vi "FT10_Fornax Power Down.vi"(10 "Auto Set Power Cluster in":T1, 11 "Message Handling Cluster in":T5={"Fornax Connected?"=refnum, "Unitherm Connected?"=refnum, "M4X Connected?"=refnum, "Unitherm Connect/Disconnect"=refnum, "Fornax Connection"=refnum, "UNITHERM Connection"="", "M4X Connection"=0, "FPGA VI Reference Out"=refnum, "PXI-7854R Connected?"=refnum, "Fornax Connect/Disconnect"=refnum, "7854 Connect/Disconnect"=refnum, "M4X Connect/Disconnect"=refnum, "Config cluster"={"Unitherm Port"="", "Simulate Values"=FALSE, "Fornax Connect Attempts"=0}, "Log Queue"=refnum, "Log Analysis Cluster - Current"={"RMS"=0.0, "Envelope Frequency"=0.0, "Peak"=0.0, "Crest Factor"=0.0, "Duty Cyle %"=0.0, "P-P"=0.0, "Frequency"=0.0, "THD"=0.0, "Postive Peak"=0.0, "Negative Peak"=0.0, "Mag_H1"=0.0, "Phase_H1"=0.0, "Mag_H3"=0.0, "Phase_H3"=0.0, "Mag_H5"=0.0, "Phase_H5"=0.0}, "Log Waveform Cluster - Current"={"t0"=timestamp(0 s since 1904-01-01), "dt"=1.0, "Y"=[]}, "Log Time"=timestamp(0 s since 1904-01-01), "Log Flag"=FALSE, "Log - Activation Settings Cluster"={"Log - Unitherm Load"="", "Log - Port"="", "Log - Mode"="", "Log - Power Level"=""}, "Log - Port Mode Cluster"={"Mono1 Cut Enum"=enum."Pure", "Mono2 Cut Enum"=enum."Pure", "Mono1 Coag Enum"=enum."Fulgerate", "Mono2 Coag Enum"=enum."Fulgerate", "Bipolar Enum"=enum."Standard"}, "Log Analysis Cluster - Diff Voltage"={"RMS"=0.0, "Envelope Frequency"=0.0, "Peak"=0.0, "Crest Factor"=0.0, "Duty Cyle %"=0.0, "P-P"=0.0, "Frequency"=0.0, "THD"=0.0, "Postive Peak"=0.0, "Negative Peak"=0.0, "Mag_H1"=0.0, "Phase_H1"=0.0, "Mag_H3"=0.0, "Phase_H3"=0.0, "Mag_H5"=0.0, "Phase_H5"=0.0}, "Log Waveform Cluster - Diff Voltage"={"t0"=timestamp(0 s since 1904-01-01), "dt"=1.0, "Y"=[]}, "Indicator Cluster"={"Mono1 - Cut Power"=refnum, "Mono1 - Coag Power"=refnum, "Mono2 - Cut Power"=refnum, "Mono2 - Coag Power"=refnum, "Bipolar Power"=refnum, "Mono1 Cut Enum"=refnum, "Mono1 Coag Enum"=refnum, "Mono2 Cut Enum"=refnum, "Mono2 Coag Enum"=refnum, "Bipolar Enum"=refnum}, "Log Power Level Cluster"={"Log Mono1 Cut Power"="", "Log Mono1 Coag Power"="", "Log Mono2 Cut Power"="", "Log Mono2 Coag Power"="", "Log Bipolar Power"=""}, "Footswitch Cluster"={"PXI-2565 reset device (boolean value)"=TRUE, "topology name"="2565/16-SPST", "PXI-2565 simulate (boolean value)"=FALSE, "PXI-2565 resource name"=""}}) -> (2 "Auto Set Power Cluster out":T1, 3 "Message Handling Cluster out":T5={"Fornax Connected?"=refnum, "Unitherm Connected?"=refnum, "M4X Connected?"=refnum, "Unitherm Connect/Disconnect"=refnum, "Fornax Connection"=refnum, "UNITHERM Connection"="", "M4X Connection"=0, "FPGA VI Reference Out"=refnum, "PXI-7854R Connected?"=refnum, "Fornax Connect/Disconnect"=refnum, "7854 Connect/Disconnect"=refnum, "M4X Connect/Disconnect"=refnum, "Config cluster"={"Unitherm Port"="COM4", "Simulate Values"=TRUE, "Fornax Connect Attempts"=0}, "Log Queue"=refnum, "Log Analysis Cluster - Current"={"RMS"=0.0, "Envelope Frequency"=0.0, "Peak"=0.0, "Crest Factor"=0.0, "Duty Cyle %"=0.0, "P-P"=0.0, "Frequency"=0.0, "THD"=0.0, "Postive Peak"=0.0, "Negative Peak"=0.0, "Mag_H1"=0.0, "Phase_H1"=0.0, "Mag_H3"=0.0, "Phase_H3"=0.0, "Mag_H5"=0.0, "Phase_H5"=0.0}, "Log Waveform Cluster - Current"={"t0"=timestamp(0 s since 1904-01-01), "dt"=1.0, "Y"=[]}, "Log Time"=timestamp(0 s since 1904-01-01), "Log Flag"=FALSE, "Log - Activation Settings Cluster"={"Log - Unitherm Load"="", "Log - Port"="", "Log - Mode"="", "Log - Power Level"=""}, "Log - Port Mode Cluster"={"Mono1 Cut Enum"=enum."Pure", "Mono2 Cut Enum"=enum."Pure", "Mono1 Coag Enum"=enum."Spray", "Mono2 Coag Enum"=enum."Spray", "Bipolar Enum"=enum."Standard"}, "Log Analysis Cluster - Diff Voltage"={"RMS"=0.0, "Envelope Frequency"=0.0, "Peak"=0.0, "Crest Factor"=0.0, "Duty Cyle %"=0.0, "P-P"=0.0, "Frequency"=0.0, "THD"=0.0, "Postive Peak"=0.0, "Negative Peak"=0.0, "Mag_H1"=0.0, "Phase_H1"=0.0, "Mag_H3"=0.0, "Phase_H3"=0.0, "Mag_H5"=0.0, "Phase_H5"=0.0}, "Log Waveform Cluster - Diff Voltage"={"t0"=timestamp(0 s since 1904-01-01), "dt"=1.0, "Y"=[]}, "Indicator Cluster"={"Mono1 - Cut Power"=refnum, "Mono1 - Coag Power"=refnum, "Mono2 - Cut Power"=refnum, "Mono2 - Coag Power"=refnum, "Bipolar Power"=refnum, "Mono1 Cut Enum"=refnum, "Mono1 Coag Enum"=refnum, "Mono2 Cut Enum"=refnum, "Mono2 Coag Enum"=refnum, "Bipolar Enum"=refnum}, "Log Power Level Cluster"={"Log Mono1 Cut Power"="", "Log Mono1 Coag Power"="", "Log Mono2 Cut Power"="", "Log Mono2 Coag Power"="", "Log Bipolar Power"=""}, "Footswitch Cluster"={"PXI-2565 reset device (boolean value)"=TRUE, "topology name"="2565/16-SPST", "PXI-2565 simulate (boolean value)"=FALSE, "PXI-2565 resource name"=""}})   [LabVIEW 2024]
doc: "Decrease power level on specified port and mode."
uses:
  Controls/Control_Message Handling Cluster.ctl
  Controls/Control_M4X Connection.ctl
  Controls/Control_PXI-7854R FPGA Reference.ctl
  Controls/Control_Config Cluster.ctl
  Controls/Control_Config Unitherm Port.ctl
  Controls/Control_Config Simulate Values.ctl
  Controls/Control_Config Fornax Connect Attempts.ctl
  Controls/Control_Log Queue.ctl
  Controls/Control_Log Cluster.ctl
  Controls/Control_Log Time.ctl
  Controls/Control_Log Waveform Cluster - Current.ctl
  Controls/Control_Log Analysis Cluster - Current.ctl
  Controls/Control_Log Activation Settings Cluster.ctl
  Controls/Control_Log Unitherm Load.ctl
  Controls/Control_Log Port.ctl
  Controls/Control_Log Mode.ctl
  Controls/Control_Log Power Level.ctl
  Controls/Control_Log Waveform Cluster - Diff Voltage.ctl
  Controls/Control_Log Analysis Cluster - Diff Voltage.ctl
  Controls/Control_Log Flag.ctl
  Controls/Control_Log Port Mode Cluster.ctl
  Controls/Control_Fornax Mono1 Cut Enum.ctl
  Controls/Control_Fornax Mono2 Cut Enum.ctl
  Controls/Control_Fornax Mono1 Coag Enum.ctl
  Controls/Control_Fornax Mono2 Coag Enum.ctl
  Controls/Control_Fornax Bipolar Enum.ctl
  Controls/Control_Indicator Cluster.ctl
  Controls/Control_Log Power Level Cluster.ctl
  Controls/Control_Log Mono1 Cut Power.ctl
  Controls/Control_Log Mono1 Coag Power.ctl
  Controls/Control_Log Mono2 Cut Power.ctl
  Controls/Control_Log Mono2 Coag Power.ctl
  Controls/Control_Log Bipolar Power.ctl
  Controls/Control_Footswitch Reset Device Bool.ctl
  <instrlib>/niSwitch/niSwitch.llb/niSwitch Topologies.ctl
  Controls/Control_Footswitch Simulate Bool.ctl
  Controls/Control_Footswitch Resource Name.ctl
  Controls/Control_Auto Set Power Cluster.ctl
  Controls/Control_Semi-Auto Port.ctl
  Controls/Control_Semi-Auto Mode.ctl
  Controls/Control_Semi-Auto Power Level.ctl
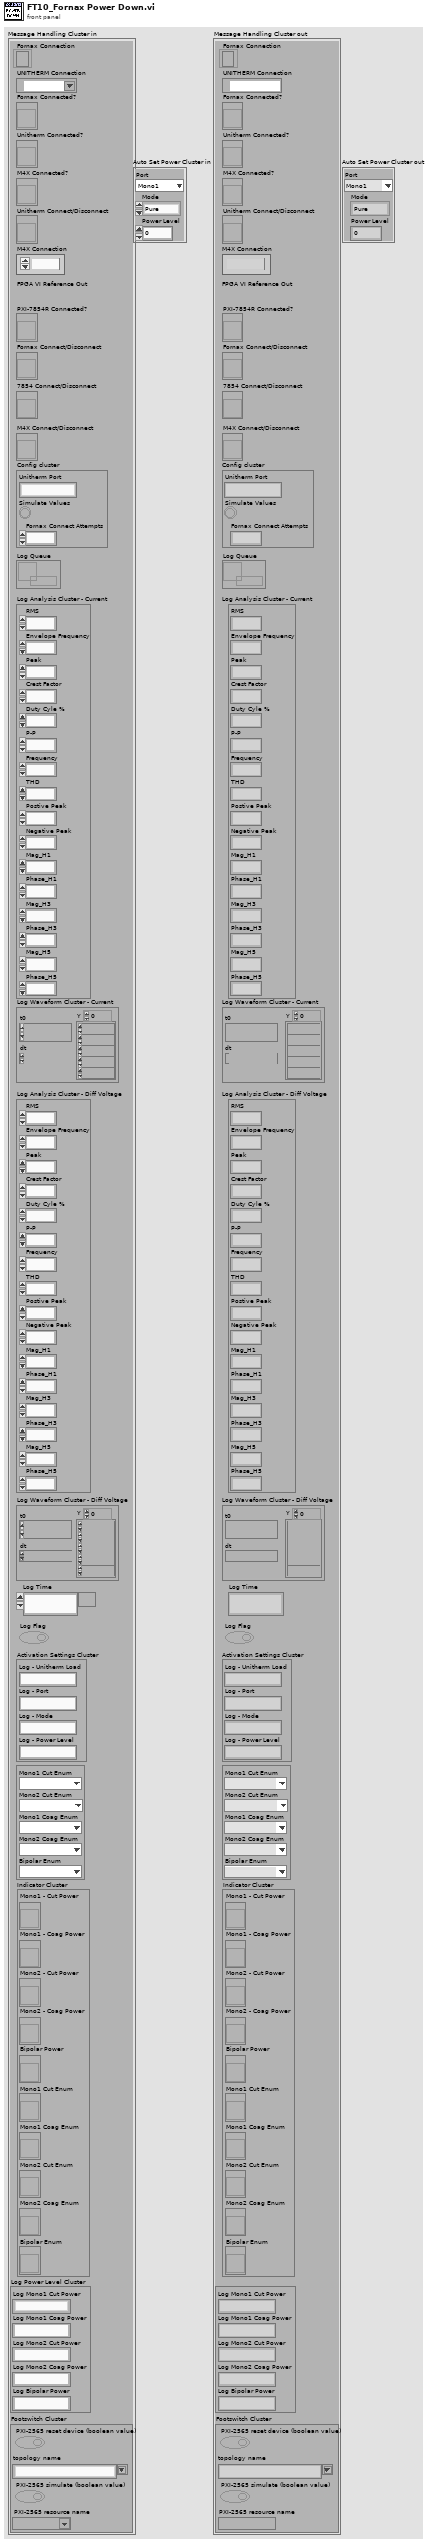
[diagram p1: front panel]
types:
  T1 = typedef "Control_Auto Set Power Cluster.ctl" = cluster{"Port":T2, "Mode":T3, "Power Level":T4}
  T2 = typedef "Control_Semi-Auto Port.ctl" = enum16{"Mono1", "Mono2", "Bipolar", "Ligasure", "Error"}
  T3 = typedef "Control_Semi-Auto Mode.ctl" = enum16{"Pure", "Blend", "Spray", "Fulgerate", "Standard", "Macro", "Precision", "Ligasure", "Error"}
  T4 = typedef "Control_Semi-Auto Power Level.ctl" = dbl
  T5 = typedef "Control_Message Handling Cluster.ctl" = cluster{"Fornax Connected?":refnum<vi>, "Unitherm Connected?":refnum<vi>, "M4X Connected?":refnum<vi>, "Unitherm Connect/Disconnect":refnum<vi>, "Fornax Connection":refnum<k5>, "UNITHERM Connection":refnum<visa-resource-name>, "M4X Connection":T6, "FPGA VI Reference Out":T7, "PXI-7854R Connected?":refnum<vi>, "Fornax Connect/Disconnect":refnum<vi>, "7854 Connect/Disconnect":refnum<vi>, "M4X Connect/Disconnect":refnum<vi>, "Config cluster":T8, "Log Queue":T12, "Log Analysis Cluster - Current":T13, "Log Waveform Cluster - Current":T14, "Log Time":T15, "Log Flag":T16, "Log - Activation Settings Cluster":T17, "Log - Port Mode Cluster":T22, "Log Analysis Cluster - Diff Voltage":T28, "Log Waveform Cluster - Diff Voltage":T29, "Indicator Cluster":T30, "Log Power Level Cluster":T31, "Footswitch Cluster":cluster{"PXI-2565 reset device (boolean value)":T37, "topology name":T38, "PXI-2565 simulate (boolean value)":T39, "PXI-2565 resource name":T40}}
  T6 = typedef "Control_M4X Connection.ctl" = u32
  T7 = typedef "Control_PXI-7854R FPGA Reference.ctl" = refnum<k20>
  T8 = typedef "Control_Config Cluster.ctl" = cluster{"Unitherm Port":T9, "Simulate Values":T10, "Fornax Connect Attempts":T11}
  T9 = typedef "Control_Config Unitherm Port.ctl" = string
  T10 = typedef "Control_Config Simulate Values.ctl" = bool
  T11 = typedef "Control_Config Fornax Connect Attempts.ctl" = i32
  T12 = typedef "Control_Log Queue.ctl" = refnum<queue>
  T13 = typedef "Control_Log Analysis Cluster - Current.ctl" = cluster{"RMS":dbl, "Envelope Frequency":dbl, "Peak":dbl, "Crest Factor":dbl, "Duty Cyle %":dbl, "P-P":dbl, "Frequency":dbl, "THD":dbl, "Postive Peak":dbl, "Negative Peak":dbl, "Mag_H1":dbl, "Phase_H1":dbl, "Mag_H3":dbl, "Phase_H3":dbl, "Mag_H5":dbl, "Phase_H5":dbl}
  T14 = typedef "Control_Log Waveform Cluster - Current.ctl" = waveform(dbl)
  T15 = typedef "Control_Log Time.ctl" = timestamp
  T16 = typedef "Control_Log Flag.ctl" = bool
  T17 = typedef "Control_Log Activation Settings Cluster.ctl" = cluster{"Log - Unitherm Load":T18, "Log - Port":T19, "Log - Mode":T20, "Log - Power Level":T21}
  T18 = typedef "Control_Log Unitherm Load.ctl" = string
  T19 = typedef "Control_Log Port.ctl" = string
  T20 = typedef "Control_Log Mode.ctl" = string
  T21 = typedef "Control_Log Power Level.ctl" = string
  T22 = typedef "Control_Log Port Mode Cluster.ctl" = cluster{"Mono1 Cut Enum":T23, "Mono2 Cut Enum":T24, "Mono1 Coag Enum":T25, "Mono2 Coag Enum":T26, "Bipolar Enum":T27}
  T23 = typedef "Control_Fornax Mono1 Cut Enum.ctl" = enum16{"Pure", "Blend"}
  T24 = typedef "Control_Fornax Mono2 Cut Enum.ctl" = enum16{"Pure", "Blend"}
  T25 = typedef "Control_Fornax Mono1 Coag Enum.ctl" = enum16{"Fulgerate", "Spray"}
  T26 = typedef "Control_Fornax Mono2 Coag Enum.ctl" = enum16{"Fulgerate", "Spray"}
  T27 = typedef "Control_Fornax Bipolar Enum.ctl" = enum16{"Standard", "Macro", "Precision"}
  T28 = typedef "Control_Log Analysis Cluster - Diff Voltage.ctl" = cluster{"RMS":dbl, "Envelope Frequency":dbl, "Peak":dbl, "Crest Factor":dbl, "Duty Cyle %":dbl, "P-P":dbl, "Frequency":dbl, "THD":dbl, "Postive Peak":dbl, "Negative Peak":dbl, "Mag_H1":dbl, "Phase_H1":dbl, "Mag_H3":dbl, "Phase_H3":dbl, "Mag_H5":dbl, "Phase_H5":dbl}
  T29 = typedef "Control_Log Waveform Cluster - Diff Voltage.ctl" = waveform(dbl)
  T30 = typedef "Control_Indicator Cluster.ctl" = cluster{"Mono1 - Cut Power":refnum<vi>, "Mono1 - Coag Power":refnum<vi>, "Mono2 - Cut Power":refnum<vi>, "Mono2 - Coag Power":refnum<vi>, "Bipolar Power":refnum<vi>, "Mono1 Cut Enum":refnum<vi>, "Mono1 Coag Enum":refnum<vi>, "Mono2 Cut Enum":refnum<vi>, "Mono2 Coag Enum":refnum<vi>, "Bipolar Enum":refnum<vi>}
  T31 = typedef "Control_Log Power Level Cluster.ctl" = cluster{"Log Mono1 Cut Power":T32, "Log Mono1 Coag Power":T33, "Log Mono2 Cut Power":T34, "Log Mono2 Coag Power":T35, "Log Bipolar Power":T36}
  T32 = typedef "Control_Log Mono1 Cut Power.ctl" = string
  T33 = typedef "Control_Log Mono1 Coag Power.ctl" = string
  T34 = typedef "Control_Log Mono2 Cut Power.ctl" = string
  T35 = typedef "Control_Log Mono2 Coag Power.ctl" = string
  T36 = typedef "Control_Log Bipolar Power.ctl" = string
  T37 = typedef "Control_Footswitch Reset Device Bool.ctl" = bool
  T38 = typedef "niSwitch Topologies.ctl" = string
  T39 = typedef "Control_Footswitch Simulate Bool.ctl" = bool
  T40 = typedef "Control_Footswitch Resource Name.ctl" = refnum<k15>
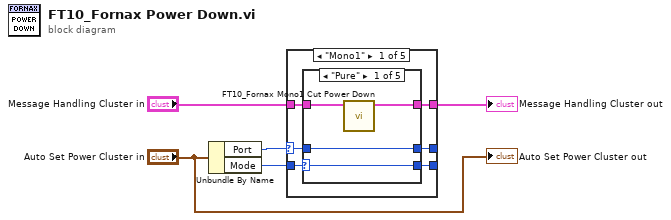
[diagram p0: block diagram]
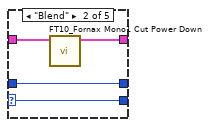
[diagram p2: hidden frame]
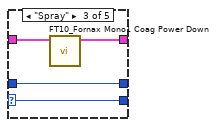
[diagram p3: hidden frame]
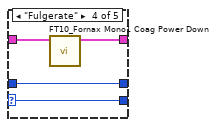
[diagram p4: hidden frame]
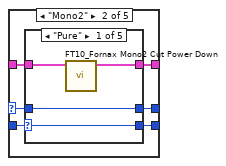
[diagram p6: hidden frame]
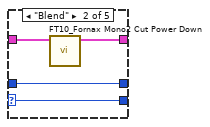
[diagram p7: hidden frame]
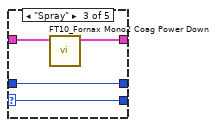
[diagram p8: hidden frame]
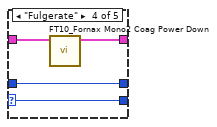
[diagram p9: hidden frame]
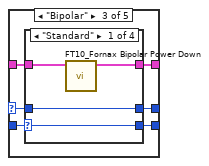
[diagram p11: hidden frame]
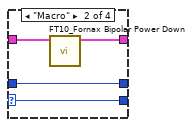
[diagram p12: hidden frame]
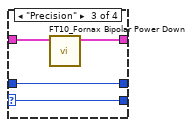
[diagram p13: hidden frame]
diagram:
  n1 = Unbundle By Name("Auto Set Power Cluster in") -> ("Port"=w2:T2, "Mode"=w1:T3)
  n2 = case shown="\"Mono1\"" w2 {
    selector: w2 -> [w7 w32 w57 w78 w90]
    tunnel: w1 -> [w11 w36 w61 w82 w94]
    tunnel: "Message Handling Cluster in" -> [w10 w35 w60 w80 w92]
    tunnel: [w9 w34 w59 w81 w93] -> w5
    tunnel: [w8 w33 w58 w79 w91] -> _
    tunnel: [w6 w31 w56 w77 w89] -> _
    frame "Mono1" {
      n3 = case shown="\"Pure\"" w11 {
        selector: w11 -> [w12 w16 w20 w24 w28]
        tunnel: w10 -> [w15 w19 w23 w27 w30]
        tunnel: [w14 w18 w22 w26 w30] -> w9
        tunnel: [w13 w17 w21 w25 w29] -> w8
        tunnel: w7 -> [w13 w17 w21 w25 w29]
        tunnel: [w12 w16 w20 w24 w28] -> w6
        frame "Pure" {
          n4 = call "FT10_Fornax Mono1 Cut Power Down.vi"("Message Handling Cluster in"=w15) -> ("Message Handling Cluster out"=w14:T5)  [unwired: 10 in]
        }
        frame "Blend" {
          n5 = call "FT10_Fornax Mono1 Cut Power Down.vi"("Message Handling Cluster in"=w19) -> ("Message Handling Cluster out"=w18:T5)  [unwired: 10 in]
        }
        frame "Spray" {
          n6 = call "FT10_Fornax Mono1 Coag Power Down.vi"("Message Handling Cluster in"=w23) -> ("Message Handling Cluster out"=w22:T5)  [unwired: 10 in]
        }
        frame "Fulgerate" {
          n7 = call "FT10_Fornax Mono1 Coag Power Down.vi"("Message Handling Cluster in"=w27) -> ("Message Handling Cluster out"=w26:T5)  [unwired: 10 in]
        }
        frame "Error", Default {
        }
      }
    }
    frame "Mono2" {
      n8 = case shown="\"Pure\"" w36 {
        selector: w36 -> [w37 w41 w45 w49 w53]
        tunnel: w35 -> [w40 w44 w48 w52 w55]
        tunnel: [w39 w43 w47 w51 w55] -> w34
        tunnel: [w38 w42 w46 w50 w54] -> w33
        tunnel: w32 -> [w38 w42 w46 w50 w54]
        tunnel: [w37 w41 w45 w49 w53] -> w31
        frame "Pure" {
          n9 = call "FT10_Fornax Mono2 Cut Power Down.vi"("Message Handling Cluster in"=w40) -> ("Message Handling Cluster out"=w39:T5)  [unwired: 10 in]
        }
        frame "Blend" {
          n10 = call "FT10_Fornax Mono2 Cut Power Down.vi"("Message Handling Cluster in"=w44) -> ("Message Handling Cluster out"=w43:T5)  [unwired: 10 in]
        }
        frame "Spray" {
          n11 = call "FT10_Fornax Mono2 Coag Power Down.vi"("Message Handling Cluster in"=w48) -> ("Message Handling Cluster out"=w47:T5)  [unwired: 10 in]
        }
        frame "Fulgerate" {
          n12 = call "FT10_Fornax Mono2 Coag Power Down.vi"("Message Handling Cluster in"=w52) -> ("Message Handling Cluster out"=w51:T5)  [unwired: 10 in]
        }
        frame "Error", Default {
        }
      }
    }
    frame "Bipolar" {
      n13 = case shown="\"Standard\"" w61 {
        selector: w61 -> [w62 w66 w70 w74]
        tunnel: w60 -> [w65 w69 w73 w76]
        tunnel: [w64 w68 w72 w76] -> w59
        tunnel: [w63 w67 w71 w75] -> w58
        tunnel: w57 -> [w63 w67 w71 w75]
        tunnel: [w62 w66 w70 w74] -> w56
        frame "Standard" {
          n14 = call "FT10_Fornax Bipolar Power Down.vi"("Message Handling Cluster in"=w65) -> ("Message Handling Cluster out"=w64:T5)  [unwired: 10 in]
        }
        frame "Macro" {
          n15 = call "FT10_Fornax Bipolar Power Down.vi"("Message Handling Cluster in"=w69) -> ("Message Handling Cluster out"=w68:T5)  [unwired: 10 in]
        }
        frame "Precision" {
          n16 = call "FT10_Fornax Bipolar Power Down.vi"("Message Handling Cluster in"=w73) -> ("Message Handling Cluster out"=w72:T5)  [unwired: 10 in]
        }
        frame "Error", Default {
        }
      }
    }
    frame "Ligasure" {
      n17 = case shown="\"Ligasure\"" w82 {
        selector: w82 -> [w83 w86]
        tunnel: [w85 w88] -> w81
        tunnel: w80 -> [w85 w88]
        tunnel: [w84 w87] -> w79
        tunnel: w78 -> [w84 w87]
        tunnel: [w83 w86] -> w77
        frame "Ligasure" {
        }
        frame "Error", Default {
        }
      }
    }
    frame "Error", Default {
      n18 = case shown="\"Error\", Default" w94 {
        selector: w94 -> [w95]
        tunnel: [w97] -> w93
        tunnel: w92 -> [w97]
        tunnel: [w96] -> w91
        tunnel: w90 -> [w96]
        tunnel: [w95] -> w89
        frame "Error", Default {
        }
      }
    }
  }
  "Message Handling Cluster out" <- w5
  "Auto Set Power Cluster out" <- "Auto Set Power Cluster in"
